vi "RehomeTensioner.vi"(11 "Buttons":bool[](array[boolean])) -> ()   [LabVIEW 2015]
uses:
  <vilib>/Rock Robotics/WPI/CAN/TalonSRX/WPI_CANTalonSRX_APIControlMode.ctl
  <vilib>/Rock Robotics/WPI/CAN/TalonSRX/WPI_CANTalonSRX_APIFeedbackSelect.ctl
panel:
  in  "Tensioner PID Gains":T1={"proportional gain (Kc)"=3.0, "integral time (Ti, min)"=0.0, "derivative time (Td, min)"=4.0}
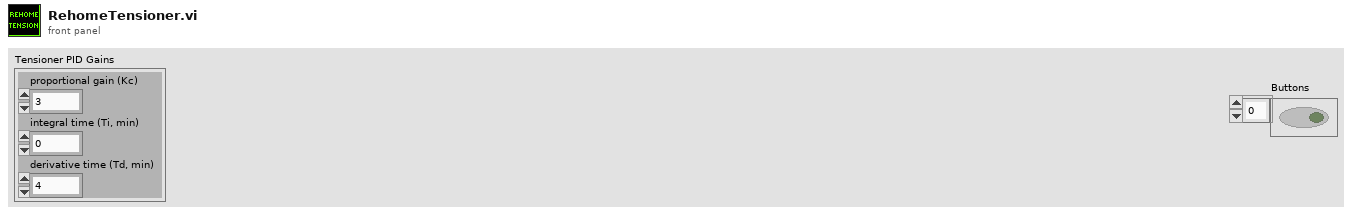
[diagram p1: front panel]
types:
  T1 = cluster{"proportional gain (Kc)":dbl, "integral time (Ti, min)":dbl, "derivative time (Td, min)":dbl}
  T2 = typedef "WPI_CANTalonSRX_APIFeedbackSelect.ctl" = enum16{"Digital Quadrature Encoder", "Analog Potentiometer", "Analog Encoder", "Count on Quad-A (Rising-Edge)", "Count on Quad-A (Falling-Edge)", "CTR Magnetic Enc (Absolute)", "CTR Magnetic Enc (Relative)", "Pulse Width"}
  T3 = typedef "WPI_CANTalonSRX_APIControlMode.ctl" = enum8{"Percent VBus", "Speed", "Position", "Slave", "Unchanged / Invalid", "Voltage Compensation", "Current", "Motion Profile"}
  T4 = typedef "WPI_SwitchDevRef.ctl" = cluster{"DevStatus":errorcluster, "DIO Channel":T5, "CntIndex":T6, "Normally Closed":bool}
  T5 = typedef "FPGA_DIOChannel.ctl" = enum8{"DIO 0", "DIO 1", "DIO 2", "DIO 3", "DIO 4", "DIO 5", "DIO 6", "DIO 7", "DIO 8", "DIO 9", "DIO MXP 0", "DIO MXP 1", "DIO MXP 2", "DIO MXP 3", "DIO MXP 4", "DIO MXP 5", "DIO MXP 6", "DIO MXP 7", "DIO MXP 8", "DIO MXP 9", "DIO MXP 10", "DIO MXP 11", "DIO MXP 12", "DIO MXP 13", "DIO MXP 14", "DIO MXP 15", "Invalid"}
  T6 = typedef "FPGA_CounterCtrSystemIndex.ctl" = enum8{"Ctr 0", "Ctr 1", "Ctr 2", "Ctr 3", "Ctr 4", "Ctr 5", "Ctr 6", "Ctr 7", "Invalid"}
  T7 = typedef "WPI_MotorControlDeviceRef.ctl" = cluster{"DeviceStatus":errorcluster, "Type":T8, "PWM":cluster{"PWM Channel":T9, "DeadBand":T10}, "CAN":cluster{"Device Number":u8, "Control Mode":T11, "Semaphore":T12, "Max Vout":dbl, "TalonSRX Control Mode":T3}, "Invert":bool}
  T8 = typedef "WPI_MotorControlType.ctl" = enum16{"PWM", "CAN", "CANTalonSRX"}
  T9 = typedef "FPGA_DIOPWMChannel.ctl" = enum8{"PWM 0", "PWM 1", "PWM 2", "PWM 3", "PWM 4", "PWM 5", "PWM 6", "PWM 7", "PWM 8", "PWM 9", "PWM MXP 0", "PWM MXP 1", "PWM MXP 2", "PWM MXP 3", "PWM MXP 4", "PWM MXP 5", "PWM MXP 6", "PWM MXP 7", "PWM MXP 8", "PWM MXP 9", "Invalid"}
  T10 = typedef "WPI_PWMDeadband.ctl" = cluster{"Name":string, "maxPositivePwm":i32, "minPositivePwm":i32, "centerPwm":i32, "maxNegativePwm":i32, "minNegativePwm":i32, "angularRange":u16}
  T11 = typedef "WPI_CANJaguar_ControlMode.ctl" = enum8{"Percent VBus", "Current", "Speed", "Position", "Voltage"}
  T12 = typedef "Semaphore RefNum" = refnum<k1>
  T13 = typedef "WPI_CANTalonSRX_GlobalStatus.ctl" = cluster{"Applied Throttle":dbl, "Module Enabled":bool, "CAN Error":errorcluster, "Closed Loop Error":dbl, "Forward Limit Switch Closed":bool, "Reverse Limit Switch Closed":bool, "Sensor Position":dbl, "Sensor Velocity":dbl, "Current":dbl, "Sticky Fault - Over Temp":bool, "Sticky Fault - Under Voltage":bool, "Sticky Fault - Forward Limit":bool, "Sticky Fault - Reverse Limit":bool, "Sticky Fault - Forward Soft Limit":bool, "Sticky Fault - Reverse Soft Limit":bool, "Brake is Enabled":bool, "Encoder Position":dbl, "Encoder Velocity":dbl, "Encoder Index Count":dbl, "Encoder A Pin State":bool, "Encoder B Pin State":bool, "Encoder Index Pin State":bool, "Analog In":dbl, "Analog In Velocity":dbl, "Temperature (C)":dbl, "Battery Voltage":dbl, "Control 5 Is Supported":bool, "Current Profile Slot Select":dbl, "Pos Div 8":bool, "Vel Div 4":bool, "Pulse Width Position":i32, "Pulse Width Velocity":i32, "Pulse Width Rise To Rise (us)":i32, "Pulse Width Rise To Fall (us)":i32, "Mot Prof Active Is Under Run":bool, "Mot Prof Active Has Under Run":bool, "Mot Prof Active Is Last":bool, "Mot Prof Active Velocity Only":bool, "Mot Prof Active Is Valid":bool, "Mot Prof Buffer Is Full":bool, "Mot Prof Active Profile Slot Select":i32, "Mot Prof NextID":i32, "Mot Prof Count":i32, "Mot Prof Active Velocity":dbl, "Mot Prof Active Position":dbl, "Mot Prof Output Enable":i32}
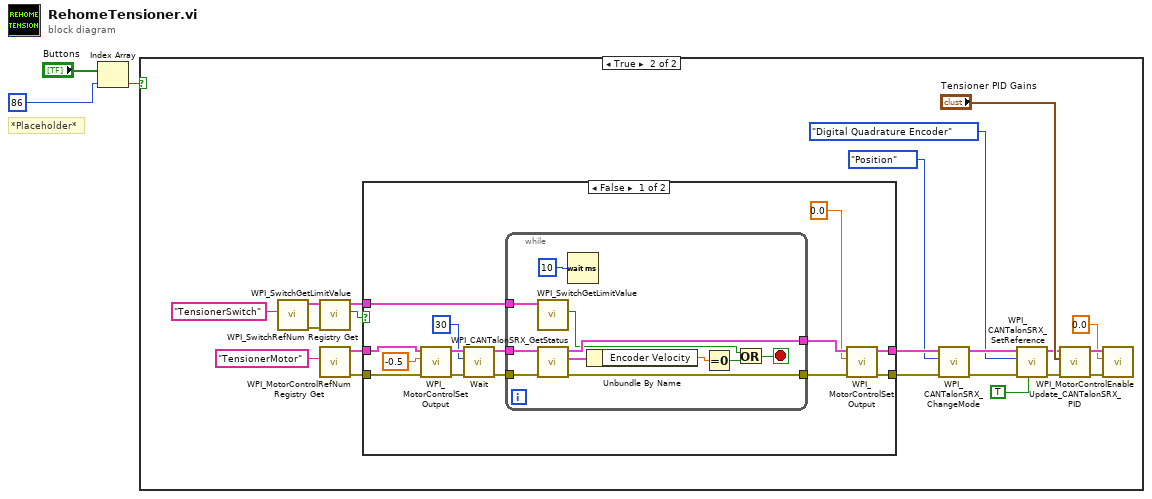
[diagram p0: block diagram]
diagram:
  # "*Placeholder*"
  n1 = Index Array(array="Buttons", index=86) -> (element=w1:bool)
  n2 = case shown="True" w1 {
    frame False {
    }
    frame True {
      n3 = call <vilib>:"WPI_SwitchRefNum Registry Get.vi"("refnum name"="TensionerSwitch") -> ("error out"=w4:errorcluster, "SwitchDevRef"=w7:T4)  [unwired: 9 in]
      n4 = call <vilib>:"WPI_SwitchGetLimitValue.vi"("error in (no error)"=w4, "SwitchDevRef"=w7) -> ("Switch Pressed"=w5:bool, "SwitchDevRef"=w6:T4)  [unwired: 7 in, 1 out]
      n5 = call <vilib>:"WPI_MotorControlRefNum Registry Get.vi"("refnum name"="TensionerMotor") -> ("error out"=w23:errorcluster, "MotorControlDevRef"=w22:T7)  [unwired: 9 in]
      n6 = case shown="False" w5 {
        tunnel: w23 -> [w38 w50]
        tunnel: w22 -> [w37 w51]
        tunnel: [w33 w51] -> w21
        tunnel: [w32 w50] -> w20
        tunnel: w6 -> [w25 _]
        frame False {
          n7 = call <vilib>:"WPI_MotorControlSetOutput.vi"("error in (no error)"=w38, "Output"=-0.5, "MotorControlDevRef"=w37) -> ("error out"=w29:errorcluster, "MotorControlDevRef"=w30:T7)  [unwired: 6 in, 1 out]
          n8 = call "Wait.vi"("error in (no error)"=w29, "milliseconds to wait"=u32 30, "MotorControlDeviceRefIn"=w30) -> ("error out"=w27:errorcluster, "MotorControlDeviceRefOut"=w28:T7)  [unwired: 7 in]
          n9 = while {
            tunnel: w25 -> [w49]
            tunnel: [w43] -> w36
            tunnel: w28 -> [w45]
            tunnel: w27 -> [w44]
            tunnel: [w42] -> w35
            stop <- w40 stop-if-true
            n10 = call <vilib>:"WPI_SwitchGetLimitValue.vi"("SwitchDevRef"=w49) -> ("Switch Pressed"=w41:bool)  [unwired: 8 in, 2 out]
            n11 = call <vilib>:"WPI_CANTalonSRX_GetStatus.vi"("error in (no error)"=w44, "CAN Talon SRX Ref"=w45) -> ("error out"=w42:errorcluster, "Talon SRX Status"=w47:T13, "CAN Talon SRX Ref"=w43:T7)  [unwired: 7 in]
            n12 = Wait (ms)(milliseconds to wait=u32 10) -> ()  [unwired: 1 out]
            n13 = Unbundle By Name(w47) -> ("Encoder Velocity"=w46:dbl)
            n14 = Equal To 0?(x=w46) -> (x = 0?=w39:bool)
            n15 = Or(x=w41, y=w39) -> (x .or. y?=w40:bool)
          }
          n16 = call <vilib>:"WPI_MotorControlSetOutput.vi"("error in (no error)"=w35, "Output"=0.0, "MotorControlDevRef"=w36) -> ("error out"=w32:errorcluster, "MotorControlDevRef"=w33:T7)  [unwired: 6 in, 1 out]
        }
        frame True {
        }
      }
      n17 = call <vilib>:"WPI_CANTalonSRX_ChangeMode.vi"("error in (no error)"=w20, "Control Mode"=WPI_CANTalonSRX_APIControlMode."Position", "CAN Talon SRX Ref"=w21) -> ("error out"=w17:errorcluster, "CAN Talon SRX Ref"=w18:T7)  [unwired: 7 in]
      n18 = call <vilib>:"WPI_CANTalonSRX_SetReference.vi"("Reverse Closed-Loop Output"=TRUE, "error in (no error)"=w17, "Feedback Reference"=WPI_CANTalonSRX_APIFeedbackSelect."Digital Quadrature Encoder", "CAN Talon SRX Ref"=w18) -> ("error out"=w13:errorcluster, "CAN Talon SRX Ref"=w14:T7)  [unwired: 6 in]
      n19 = call "Update_CANTalonSRX_PID.vi"("error in (no error)"=w13, "PID Gains"="Tensioner PID Gains", "CAN Talon SRX Ref"=w14) -> ("error out"=w11:errorcluster, "CAN Talon SRX Ref Out"=w12:T7)  [unwired: 7 in]
      n20 = call <vilib>:"WPI_MotorControlEnable.vi"("error in (no error)"=w11, "Encoder Initial Position"=0.0, "CAN MotorDevRef"=w12) -> ()  [unwired: 7 in, 2 out]
    }
  }
